vi "NIMS_TargetSyntax_BIFTableToVariant.vi"(1 "BIFTable in":refnum<class "HashTable.lvclass">) -> (0 "BIFTable out":variant)   [LabVIEW 2021]
uses:
  <vilib>/imath/engines/lvmath2/StdLib/HashTable.llb/HashTable.lvclass
  <vilib>/imath/engines/lvmath2/MathScriptCompiler/TargetSyntax/NIMS_TargetSyntax_BIFSignature.ctl
  <vilib>/imath/engines/lvmath2/MathScriptCompiler/TargetSyntax/NIMS_TargetSyntax_BIFInfo.ctl
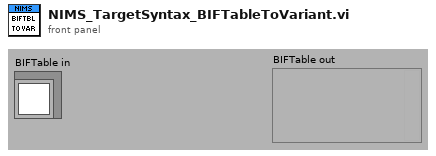
[diagram p1: front panel]
types:
  T1 = typedef "NIMS_TargetSyntax_BIFSignature.ctl" = cluster{"Function":string, "BIFInfo(s)":T2[]}
  T2 = typedef "NIMS_TargetSyntax_BIFInfo.ctl" = cluster{"Number of inputs":i32, "Number of outputs requested":i32, "Line number":u32, "Column number":u32}
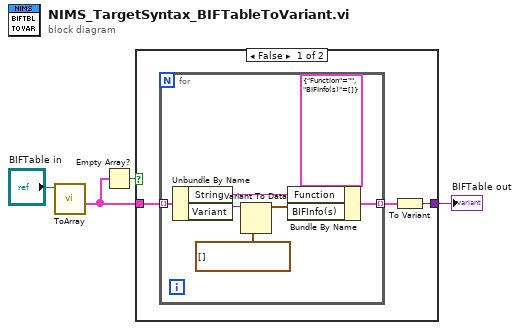
[diagram p0: block diagram]
diagram:
  n1 = call <vilib>:"ToArray.vi"("HashTable in"="BIFTable in") -> ("Array"=w1:cluster{"String":string, "Variant":variant}[])  [unwired: 10 out]
  n2 = Empty Array?(array=w1) -> (empty?=w2:bool)
  n3 = case shown="False" w2 {
    tunnel: w1 -> [w7 _]
    tunnel: [w5 _] -> w3
    frame False {
      n4 = for {
        tunnel: w7 -> [w14] mode=indexing
        tunnel: [w8] -> w6 mode=indexing
        n5 = Unbundle By Name(w14) -> ("String"=w10:string, "Variant"=w13:variant)
        n6 = Variant To Data(type=T2[] [], Variant=w13) -> (data=w9:T2[])  [unwired: 1 in, 1 out]
        n7 = Bundle By Name(cluster=T1 {"Function"="", "BIFInfo(s)"=[]} ("BIFSignature"), "Function"=w10, "BIFInfo(s)"=w9) -> (w8:T1)
      }
      n8 = To Variant(anything=w6) -> (Variant=w5:variant)
    }
    frame True {
    }
  }
  "BIFTable out" <- w3
